vi "_TCP Msg Read.vi"(7 "RT":bool, 8 "error in":errorcluster, 10 "timeout ms (10000)":i32=10000, 11 "connection ID":refnum<k5>) -> (0 "error out":errorcluster, 1 "Read Timeout":bool, 2 "Packet Info":T1={"Packet Signature"="", "Sequence Number"=0, "Command"=enum."xml Set LC Input Logic", "Data Message Size"=0, "Data Message Size"="", "Data Message"="", "Error Message Size"=0, "Error Message Size"="", "Error Message"="", "Checksum"=0, "Error Message"={"status"=FALSE, "code"=0, "source"=""}, "Command ID"=""}, 3 "connection ID out":refnum<k5>)   [LabVIEW 2015]
doc: "Reads an incoming package of data from a remote host via TCP/IP. This VI parses the package and extracts the data name and type as described in the meta data.\n\nFor the package to be parsed correctly, the meta data must be consistent in both the sender and the receiver. The data is packaged based on the existing meta data on the sender. Inconsistent meta data will result in inconsistent data parsing.\nUse the \"Read Meta\" and \"Write Meta\" VIs to ensure that both client and server have the same meta data.\n\nThe data is returned as a string. It is the responsibility of the user to cast it to the appropriate type before usage."
uses:
  Types/TCP Packet Info.ctl
  Types/_RT Command.ctl
  Types/TCP Packet Parsing State Machine.ctl
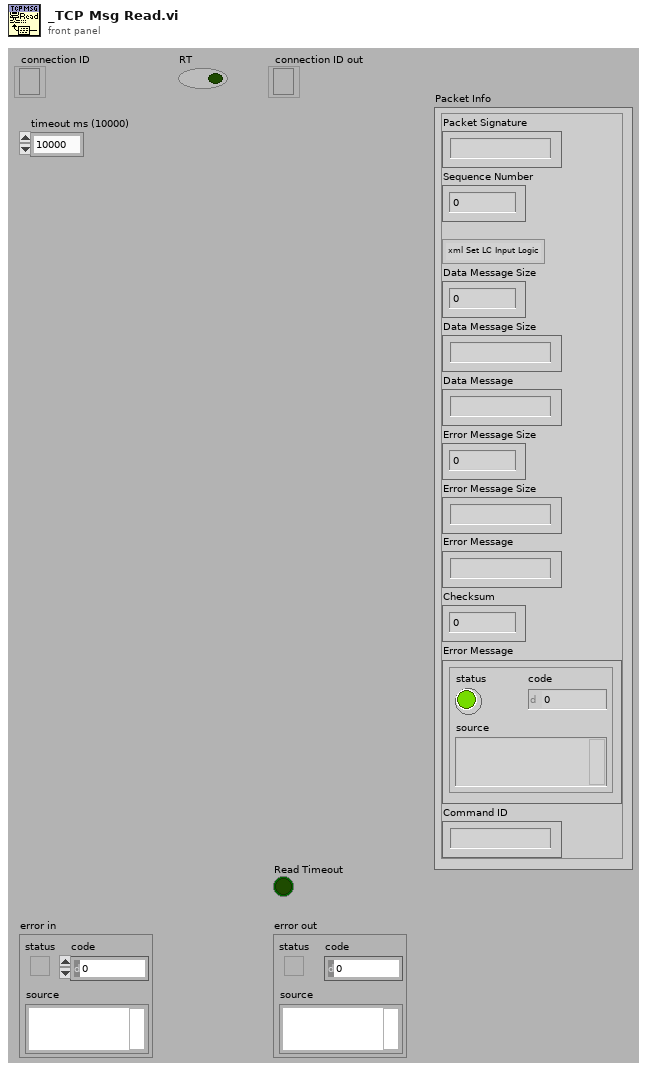
[diagram p1: front panel]
types:
  T1 = typedef "TCP Packet Info.ctl" = cluster{"Packet Signature":string, "Sequence Number":i32, "Command":T2, "Data Message Size":u32, "Data Message Size":string, "Data Message":string, "Error Message Size":u32, "Error Message Size":string, "Error Message":string, "Checksum":u32, "Error Message":errorcluster, "Command ID":string}
  T2 = typedef "_RT Command.ctl" = enum16{"xml Start Run", "xml Start Actual Run", "xml Stop Run", "xml Runtime Update", "xml Get Status", "xml Get Table", "xml Set Table", "xml Get Configuration", "xml System Status", "xml Set LC Input Logic", "xml Get Data", "xml Get Info", "Start", "StartActualRun", "Stop", "Runtime Update", "Get Data", "Get Info", "Get Status", "Get Param", "Get Config", "Get Table", "Read ADC", "Set Oscillator", "Update Config", "Update Table", "Set All Pol", "Set Pol and DC", "Set Max Mass", "Toggle RP", "Toggle EL", "Set PIC", "Initialize Turbo", "Send Turbo Comm", "Close Turbo", "P1", "P2", "P3", "Send Serial", "Set LC Out", "Get LC In", "Read VAC", "Test Table", "Toggle Power", "Get Startup", "Set Startup", "Get ADC Table", "Set ADC Table", "Get Brief Status", "Get Detail Status", "Auxiliary Update", "Set CC Logics", "Set CC Input Logics", "Ignore Error", "invalid"}
  T3 = typedef "TCP Packet Parsing State Machine.ctl" = enum16{"Packet Signature", "Sequence Number", "Command ID", "Data Message Size", "Data Message", "Error Message Size", "Error Message", "Checksum", "Invalid Packet Structure"}
  T4 = enum16{"big-endian, network order", "native, host order", "little-endian"}
  T5 = enum16{"Standard", "Buffered", "CRLF", "Immediate"}
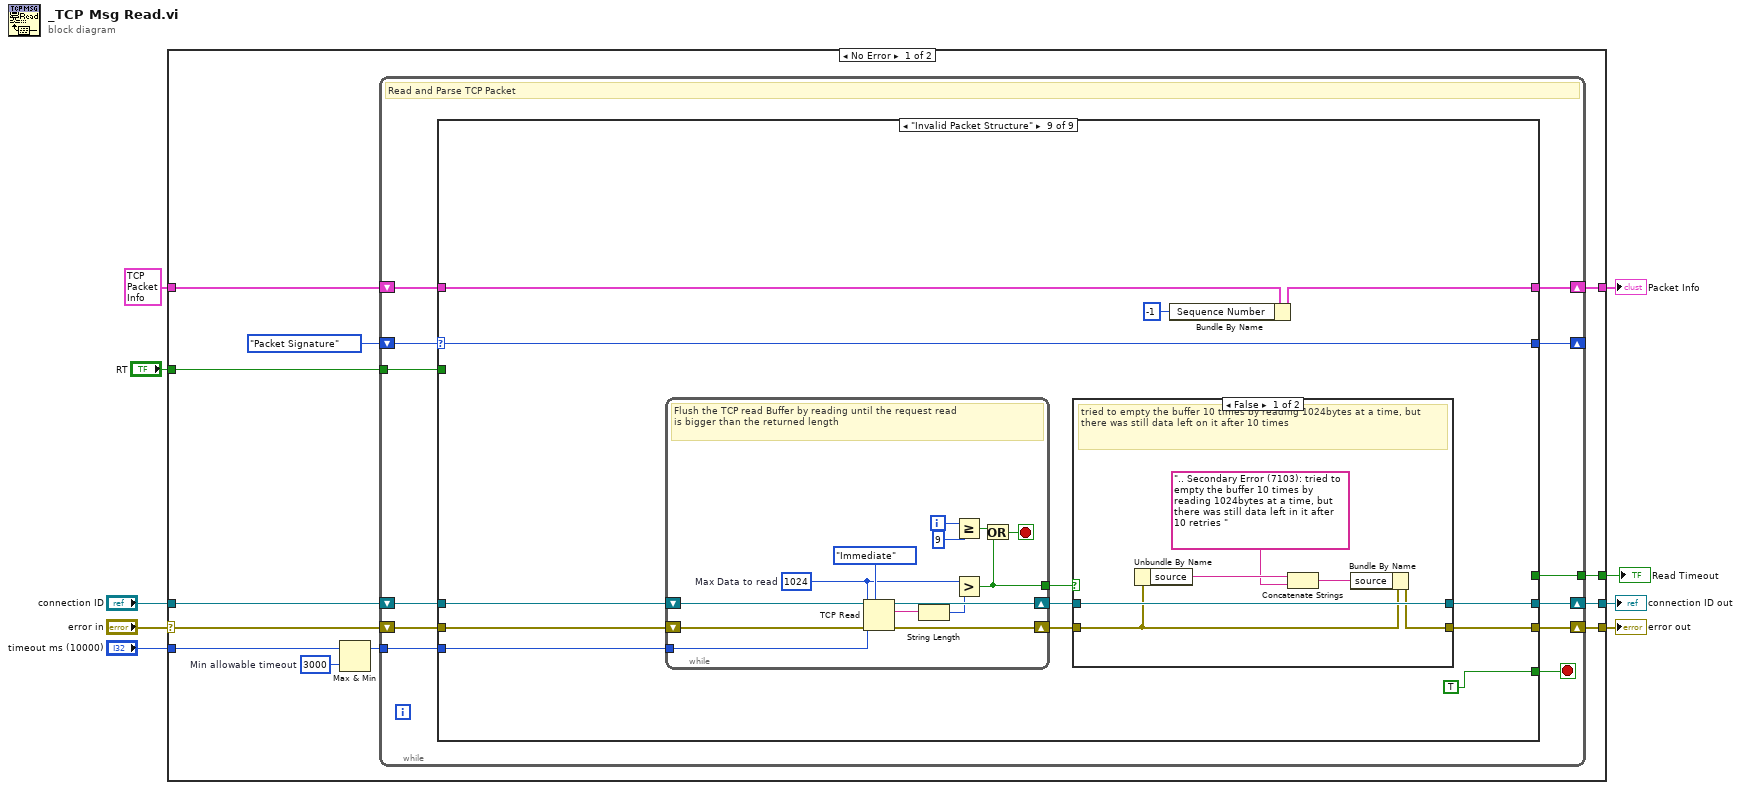
[diagram p0: block diagram]
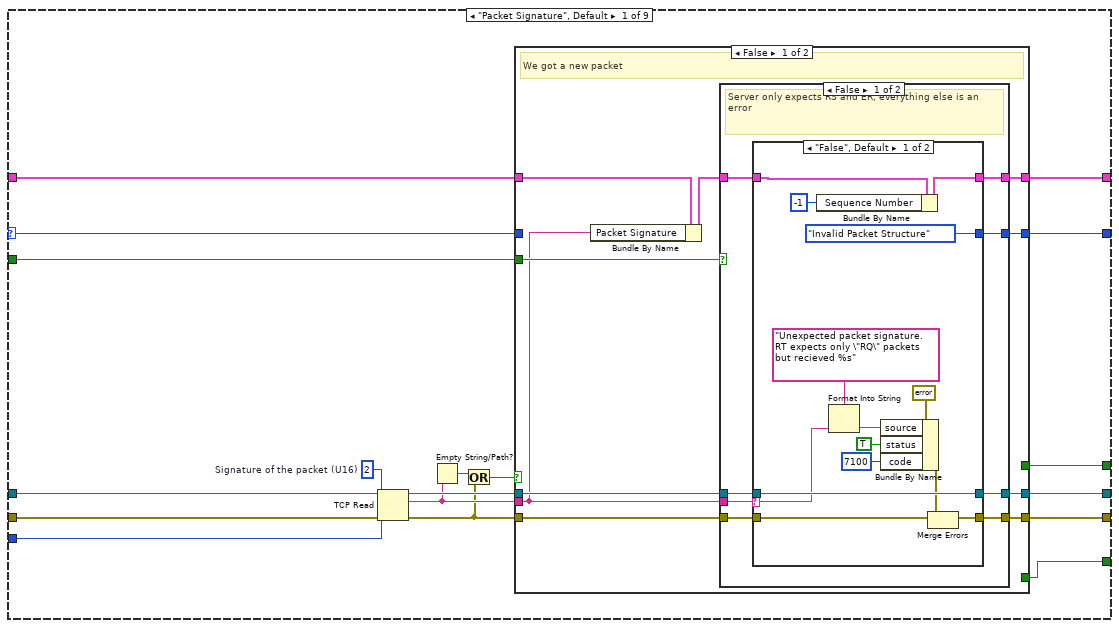
[diagram p2: hidden frame]
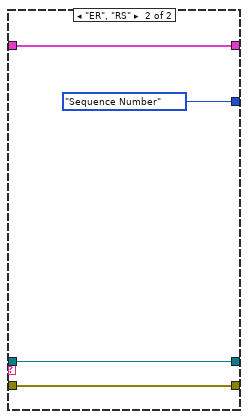
[diagram p3: hidden frame]
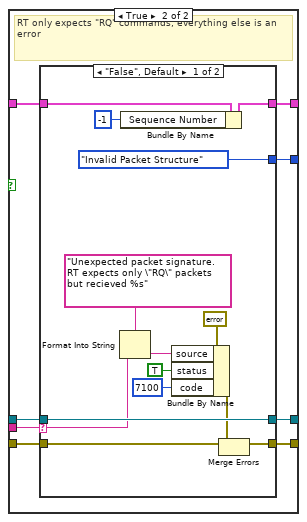
[diagram p4: hidden frame]
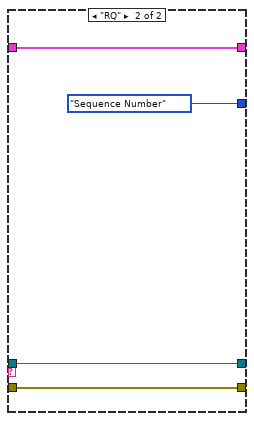
[diagram p5: hidden frame]
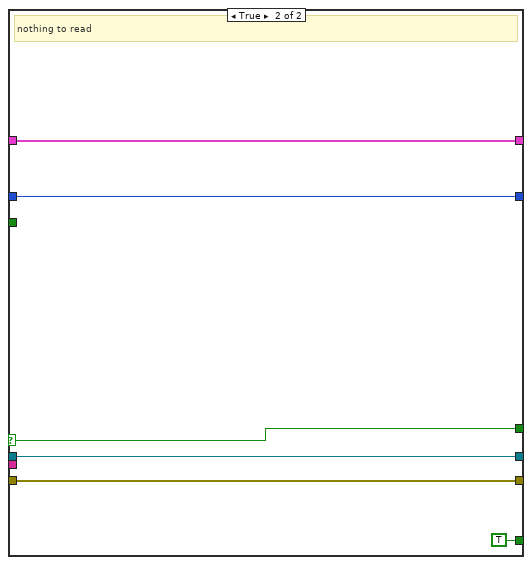
[diagram p6: hidden frame]
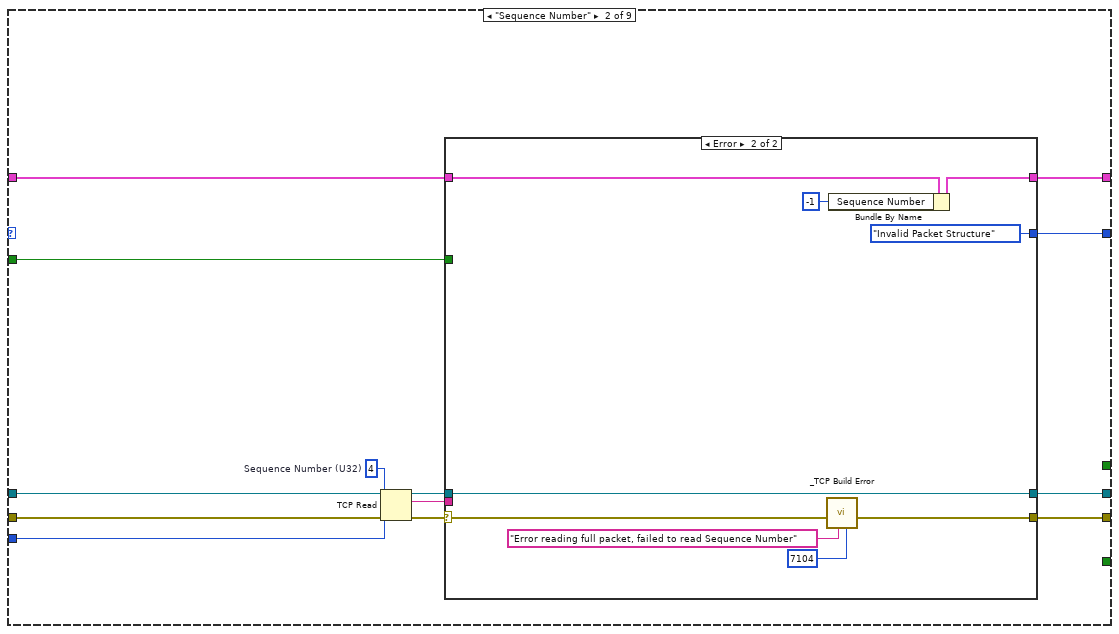
[diagram p7: hidden frame]
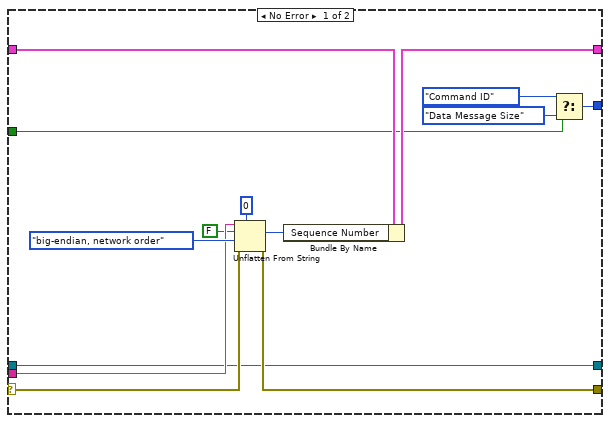
[diagram p8: hidden frame]
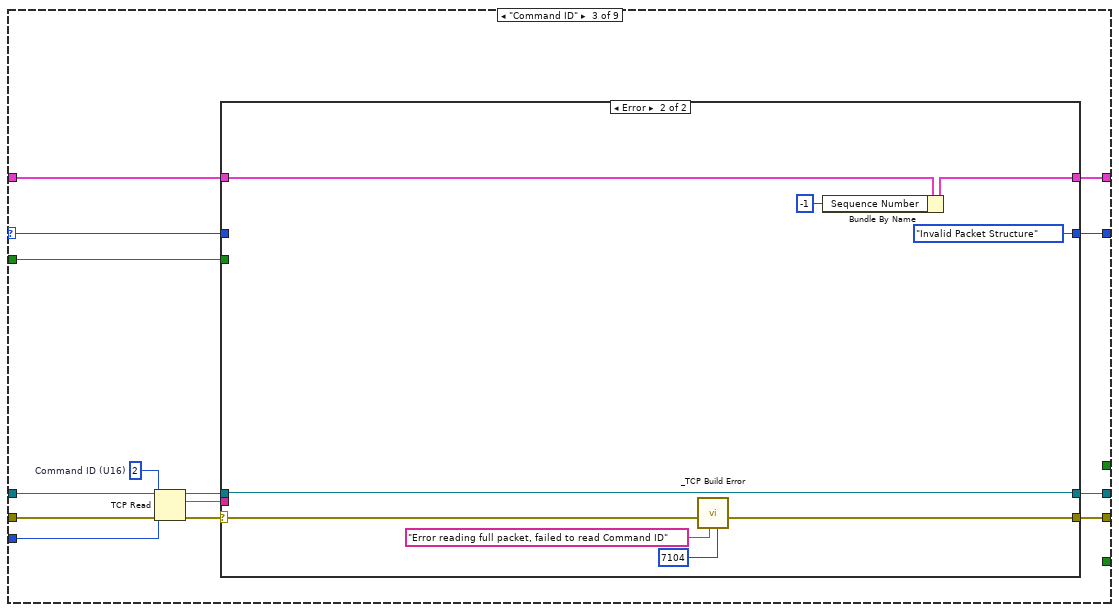
[diagram p9: hidden frame]
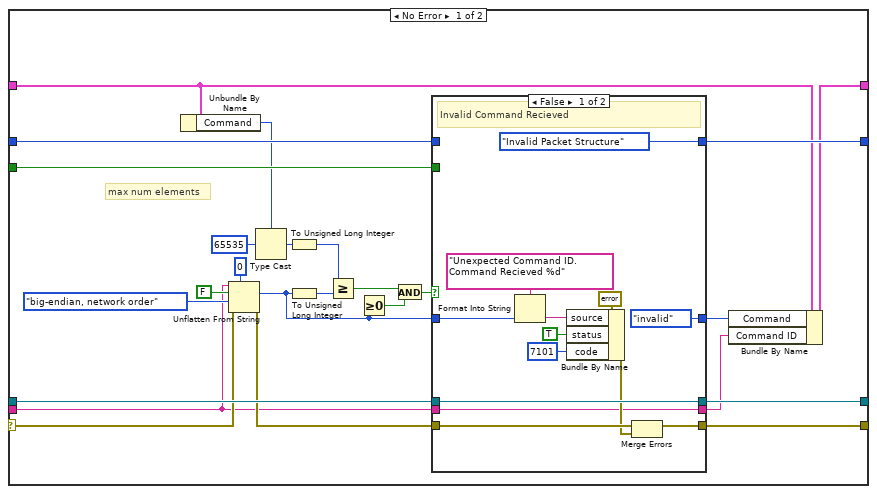
[diagram p10: hidden frame]
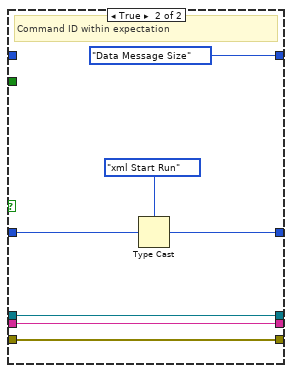
[diagram p11: hidden frame]
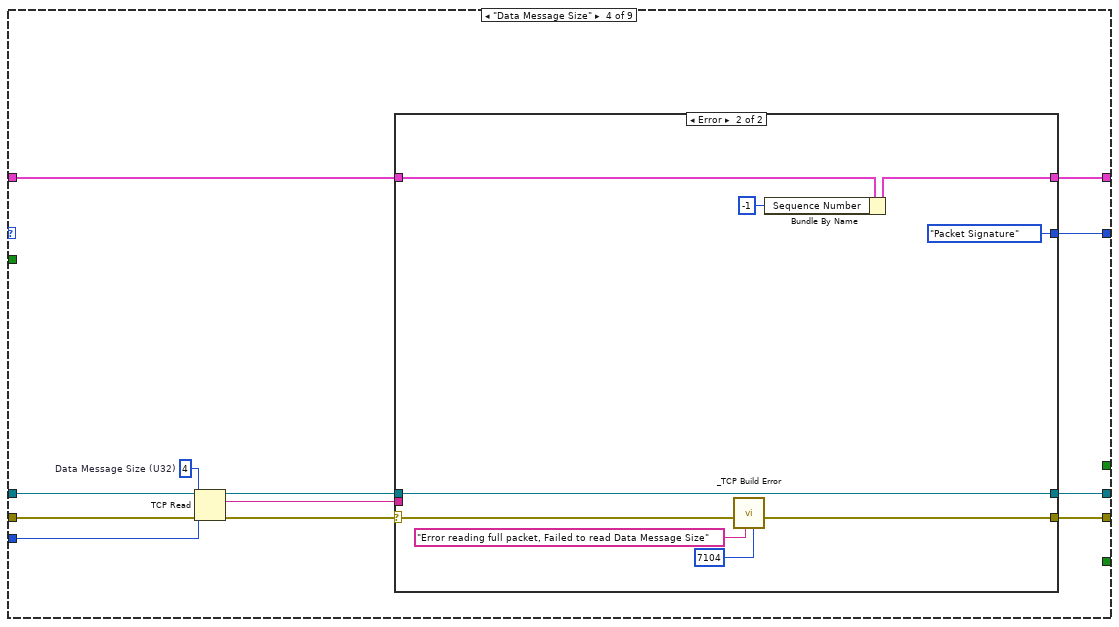
[diagram p12: hidden frame]
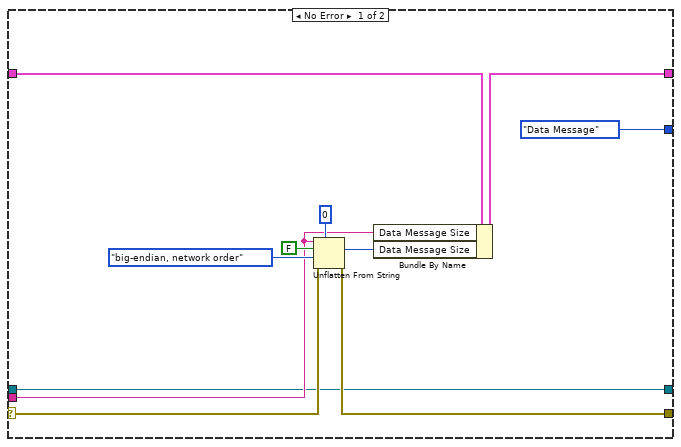
[diagram p13: hidden frame]
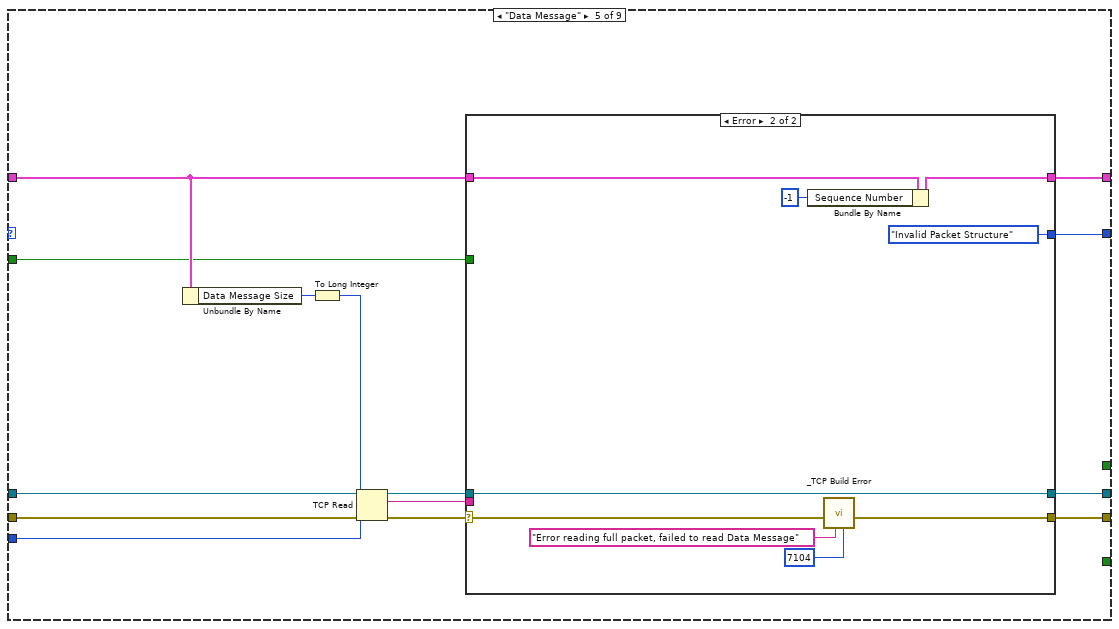
[diagram p14: hidden frame]
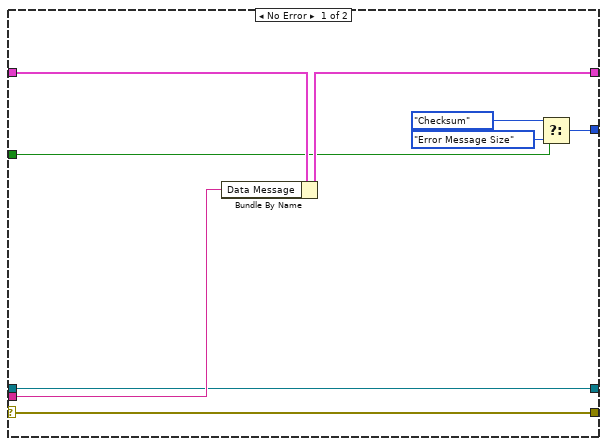
[diagram p15: hidden frame]
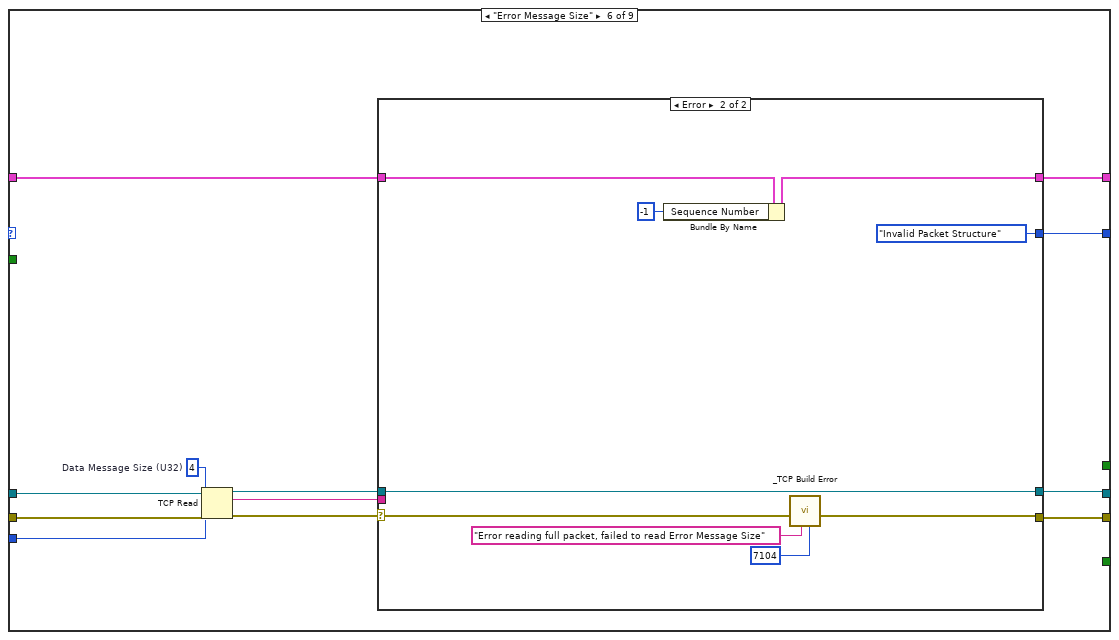
[diagram p16: hidden frame]
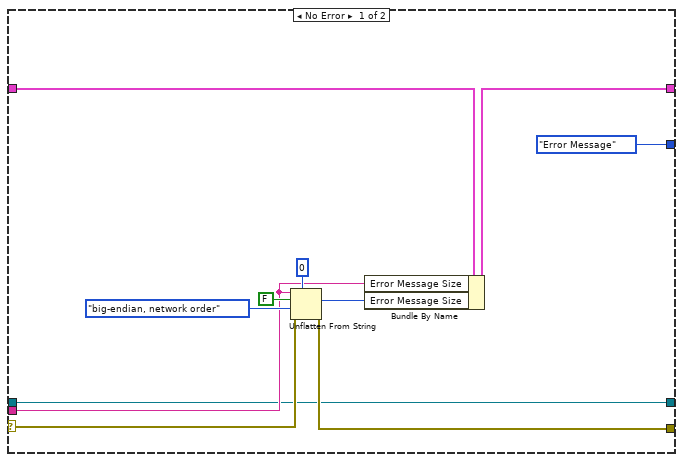
[diagram p17: hidden frame]
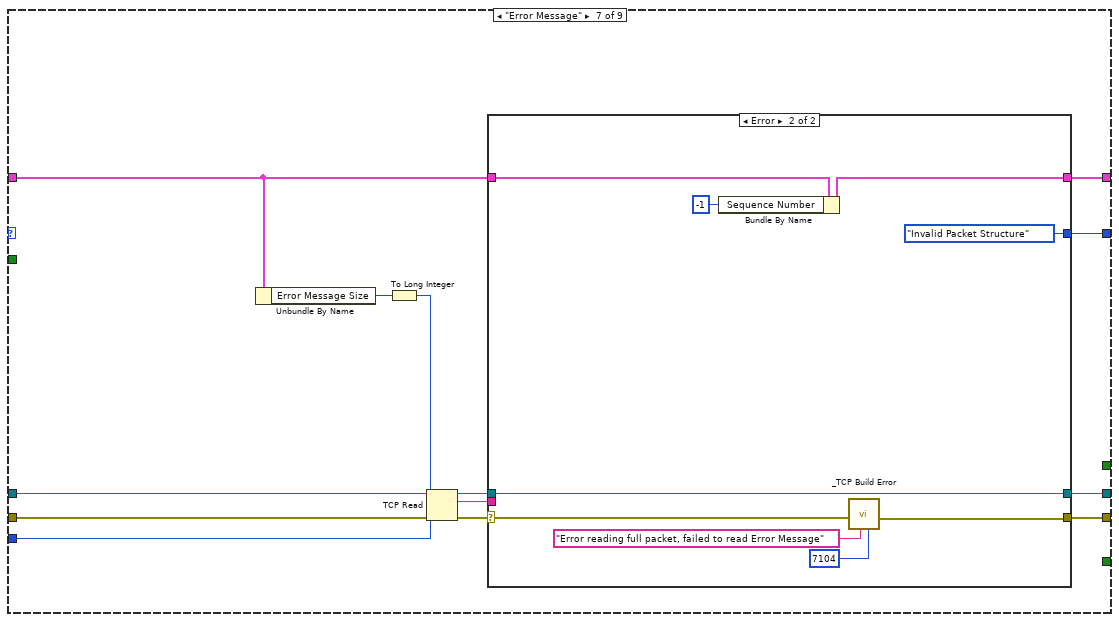
[diagram p18: hidden frame]
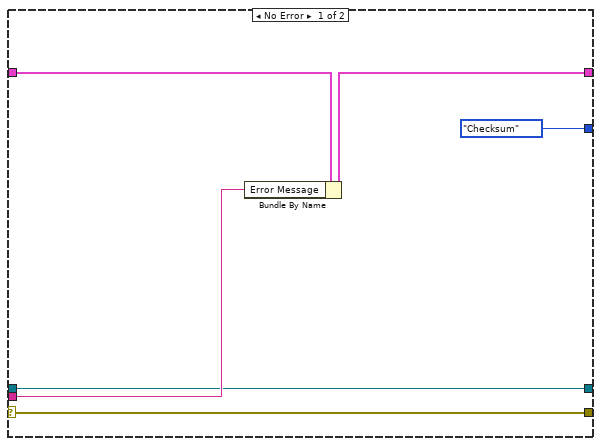
[diagram p19: hidden frame]
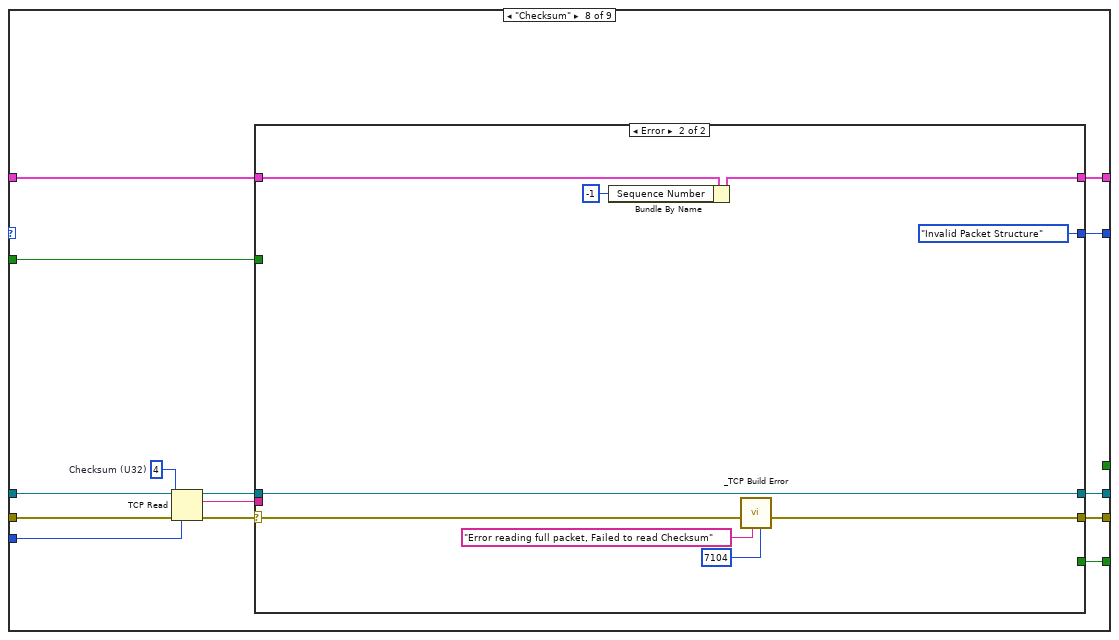
[diagram p20: hidden frame]
diagram:
  n1 = case shown="No Error" "error in" {
    selector: "error in" -> [w19 w453]
    tunnel: T1 {"Packet Signature"="", "Sequence Number"=0, "Command"=enum."xml Set LC Input Logic", "Data Message Size"=0, "Data Message Size"="", "Data Message"="", "Error Message Size"=0, "Error Message Size"="", "Error Message"="", "Checksum"=0, "Error Message"={"status"=FALSE, "code"=0, "source"=""}, "Command ID"=""} ("Packet Info") -> [w21 w452]
    tunnel: "connection ID" -> [w20 w454]
    tunnel: "timeout ms (10000)" -> [w18 _]
    tunnel: "RT" -> [w17 _]
    tunnel: [w16 w454] -> w5
    tunnel: [w15 w453] -> w4
    tunnel: [w14 w452] -> w3
    tunnel: [w10 _] -> w1
    frame No Error {
      w12 = 3000  # Min allowable timeout
      n2 = Max & Min(x=w18, y=w12) -> (max(x,y)=w11:i32)  [unwired: 1 out]
      n3 = while {
        shift-right: [w32] -> w14
        shift-left: w21 -> [w33]
        shift-right: [w27] -> w16
        shift-left: w20 -> [w31]
        shift-right: [w28] -> w15
        shift-left: w19 -> [w30]
        tunnel: w11 -> [w29]
        tunnel: w17 -> [w26]
        shift-right: [w25] -> _
        shift-left: TCP_Packet_Parsing_State_Machine."Packet Signature" ("Packet Structure") -> [w23]
        tunnel: [w22] -> w10
        stop <- w24 stop-if-true
        # "Read and Parse TCP Packet"
        n4 = case shown="\"Invalid Packet Structure\"" w23 {
          selector: w23 -> [w39 _ w164 _ _ _ _ _ w428]
          tunnel: w33 -> [w41 w132 w159 w231 w264 w295 w326 w355 w418]
          tunnel: [w43 w127 w161 w230 w263 w294 w325 w357 w417] -> w32
          tunnel: w31 -> [w50 w130 w167 w233 w268 w297 w328 w361 w426]
          tunnel: w30 -> [w49 w129 w166 w234 w269 w298 w329 w359 w427]
          tunnel: w29 -> [w47 w128 w165 w232 w267 w296 w327 w360 w425]
          tunnel: [w45 w122 w157 w227 w259 w291 w321 w352 w420] -> w28
          tunnel: [w44 w121 w162 w225 w256 w288 w323 w354 w422] -> w27
          tunnel: w26 -> [w46 w126 w160 _ w260 _ _ w348 _]
          tunnel: [w42 w125 w163 w229 w261 w293 w324 w356 w428] -> w25
          tunnel: [w38 _ _ _ _ _ _ w351 TRUE] -> w24
          tunnel: [w37 _ _ _ _ _ _ _ _] -> w22
          frame "Packet Signature", Default {
            w51 = 2  # Signature of the packet (U16)
            # "Packet Header"
            n5 = TCP Read(connection ID=w50, bytes to read=w51, error in (no error)=w49, 9:w47) -> (connection ID out=w48:refnum<k5>, data out=w40:string, error out=w34:errorcluster)  [unwired: 1 out]
            n6 = Empty String/Path?(string/path=w40) -> (empty?=w36:bool)
            n7 = Or(x=w36, y=w34) -> (x .or. y?=w35:bool)
            n8 = case shown="False" w35 {
              selector: w35 -> [_ w114]
              tunnel: w48 -> [w61 w117]
              tunnel: w34 -> [w60 w116]
              tunnel: w46 -> [w59 _]
              tunnel: [w58 w116] -> w45
              tunnel: [w57 w117] -> w44
              tunnel: [w56 w119] -> w43
              tunnel: [w55 w118] -> w42
              tunnel: w41 -> [w54 w119]
              tunnel: w40 -> [w52 _]
              tunnel: w39 -> [_ w118]
              tunnel: [_ TRUE] -> w38
              tunnel: [_ w114] -> w37
              frame False {
                # "We got a new packet"
                n9 = Bundle By Name(cluster=w54, "Packet Signature"=w52) -> (w53:T1)
                n10 = case shown="False" w59 {
                  tunnel: w52 -> [w68 w90]
                  tunnel: w61 -> [w67 w95]
                  tunnel: w60 -> [w69 w94]
                  tunnel: [w66 w93] -> w57
                  tunnel: [w65 w92] -> w58
                  tunnel: w53 -> [w62 w88]
                  tunnel: [w63 w89] -> w56
                  tunnel: [w64 w91] -> w55
                  frame False {
                    # "Server only expects RS and ER, everything else is an error"
                    n11 = case shown="\"False\", Default" w68 {
                      selector: w68 -> [w73 _]
                      tunnel: w69 -> [w75 w86]
                      tunnel: w67 -> [w83 w87]
                      tunnel: [w83 w87] -> w66
                      tunnel: [w76 w86] -> w65
                      tunnel: [TCP_Packet_Parsing_State_Machine."Invalid Packet Structure" ("Packet Structure") TCP_Packet_Parsing_State_Machine."Sequence Number" ("Packet Structure")] -> w64
                      tunnel: [w70 w84] -> w63
                      tunnel: w62 -> [w71 w84]
                      frame "False", Default {
                        n12 = Bundle By Name(cluster=w71, "Sequence Number"=-1) -> (w70:T1)
                        n13 = Format Into String(format string="Unexpected packet signature. RT expects only \"RQ\" packets but recieved %s" ("source"), w73) -> (resulting string=w78:string)  [unwired: 2 in, 1 out]
                        n14 = Bundle By Name(cluster=errorcluster {"status"=FALSE, "code"=0, "source"=""} ("error IO"), "source"=w78, "status"=TRUE, "code"=7100) -> (w77:errorcluster)
                        n15 = Merge Errors(w75, w77) -> (w76:errorcluster)
                      }
                      frame "ER", "RS" {
                      }
                    }
                  }
                  frame True {
                    # "RT only expects \"RQ\" commands, everything else is an error"
                    n16 = case shown="\"False\", Default" w90 {
                      selector: w90 -> [w104 _]
                      tunnel: w95 -> [w109 w113]
                      tunnel: w94 -> [w101 w112]
                      tunnel: [w109 w113] -> w93
                      tunnel: [w100 w112] -> w92
                      tunnel: [TCP_Packet_Parsing_State_Machine."Invalid Packet Structure" ("Packet Structure") TCP_Packet_Parsing_State_Machine."Sequence Number" ("Packet Structure")] -> w91
                      tunnel: [w97 w110] -> w89
                      tunnel: w88 -> [w98 w110]
                      frame "False", Default {
                        n17 = Format Into String(format string="Unexpected packet signature. RT expects only \"RQ\" packets but recieved %s" ("source"), w104) -> (resulting string=w103:string)  [unwired: 2 in, 1 out]
                        n18 = Bundle By Name(cluster=w98, "Sequence Number"=-1) -> (w97:T1)
                        n19 = Bundle By Name(cluster=errorcluster {"status"=FALSE, "code"=0, "source"=""} ("error IO"), "source"=w103, "status"=TRUE, "code"=7100) -> (w102:errorcluster)
                        n20 = Merge Errors(w101, w102) -> (w100:errorcluster)
                      }
                      frame "RQ" {
                        # "\"RQ\""
                      }
                    }
                  }
                }
              }
              frame True {
                # "nothing to read"
              }
            }
          }
          frame "Sequence Number" {
            w131 = 4  # Sequence Number (U32)
            n21 = TCP Read(connection ID=w130, bytes to read=w131, error in (no error)=w129, 9:w128) -> (connection ID out=w120:refnum<k5>, data out=w123:string, error out=w124:errorcluster)  [unwired: 1 out]
            n22 = case shown="Error" w124 {
              selector: w124 -> [w140 w153]
              tunnel: w132 -> [w146 w148]
              tunnel: [w145 w147] -> w127
              tunnel: w126 -> [w144 _]
              tunnel: [w142 TCP_Packet_Parsing_State_Machine."Invalid Packet Structure" ("f")] -> w125
              tunnel: w123 -> [w136 _]
              tunnel: [w134 w152] -> w122
              tunnel: [w133 w155] -> w121
              tunnel: w120 -> [w133 w155]
              frame No Error {
                n23 = Unflatten From String(type=0, binary string=w136, data includes array or string size? (T)=FALSE, byte order (0:big-endian, network order)=T4."big-endian, network order", error in (no error)=w140) -> (value=w137:i32, error out=w134:errorcluster)  [unwired: 1 out]
                n24 = Bundle By Name(cluster=w146, "Sequence Number"=w137) -> (w145:T1)
                n25 = Select(t=TCP_Packet_Parsing_State_Machine."Command ID" ("Packet Structure"), s=w144, f=TCP_Packet_Parsing_State_Machine."Data Message Size") -> (s? t:f=w142:T3)
              }
              frame Error {
                n26 = call "_TCP Build Error.vi"("code"=7104, "Error"="Error reading full packet, failed to read Sequence Number", "error in (no error)"=w153) -> ("error out"=w152:errorcluster)  [unwired: 8 in]
                n27 = Bundle By Name(cluster=w148, "Sequence Number"=-1) -> (w147:T1)
              }
            }
          }
          frame "Command ID" {
            w168 = 2  # Command ID (U16)
            n28 = TCP Read(connection ID=w167, bytes to read=w168, error in (no error)=w166, 9:w165) -> (connection ID out=w169:refnum<k5>, data out=w156:string, error out=w158:errorcluster)  [unwired: 1 out]
            n29 = case shown="Error" w158 {
              selector: w158 -> [w175 w221]
              tunnel: w169 -> [w190 w220]
              tunnel: w164 -> [w186 _]
              tunnel: [w185 TCP_Packet_Parsing_State_Machine."Invalid Packet Structure" ("Packet Structure")] -> w163
              tunnel: [w184 w220] -> w162
              tunnel: [w183 w215] -> w161
              tunnel: w160 -> [w181 _]
              tunnel: w159 -> [w180 w216]
              tunnel: [w172 w219] -> w157
              tunnel: w156 -> [w170 _]
              frame No Error {
                # "max num elements"
                n30 = Unbundle By Name(w180) -> ("Command"=w179:T2)
                n31 = Unflatten From String(type=u16 0, binary string=w170, data includes array or string size? (T)=FALSE, byte order (0:big-endian, network order)=T4."big-endian, network order", error in (no error)=w175) -> (value=w173:u16, error out=w174:errorcluster)  [unwired: 1 out]
                n32 = Type Cast(type=w179, x=u16 65535 ("default value 1")) -> (*(type *) &x=w189:T2)
                n33 = To Unsigned Long Integer(number=w189) -> (unsigned 32bit integer=w187:u32)
                n34 = To Unsigned Long Integer(number=w173) -> (unsigned 32bit integer=w191:u32)
                n35 = Greater Or Equal?(x=w187, y=w191) -> (x >= y?=w192:bool)
                n36 = Greater Or Equal To 0?(x=w173) -> (x >= 0?=w194:bool)
                n37 = And(x=w192, y=w194) -> (x .and. y?=w193:bool)
                n38 = case shown="False" w193 {
                  tunnel: [w198 w214] -> w172
                  tunnel: w174 -> [w200 w214]
                  tunnel: [w207 w213] -> w184
                  tunnel: w190 -> [w207 w213]
                  tunnel: w173 -> [w201 w212]
                  tunnel: [_RT_Command."invalid" ("Command") w211] -> w182
                  tunnel: w186 -> [_ _]
                  tunnel: [TCP_Packet_Parsing_State_Machine."Invalid Packet Structure" ("Packet Structure") TCP_Packet_Parsing_State_Machine."Data Message Size" ("Packet Structure")] -> w185
                  tunnel: w181 -> [_ _]
                  tunnel: [w195 w208] -> w171
                  tunnel: w170 -> [w195 w208]
                  frame False {
                    # "Invalid Command Recieved"
                    n39 = Format Into String(format string="Unexpected Command ID. Command Recieved %d" ("source"), w201) -> (resulting string=w202:string)  [unwired: 2 in, 1 out]
                    n40 = Bundle By Name(cluster=errorcluster {"status"=FALSE, "code"=0, "source"=""} ("error IO"), "source"=w202, "status"=TRUE, "code"=7101) -> (w199:errorcluster)
                    n41 = Merge Errors(w200, w199) -> (w198:errorcluster)
                  }
                  frame True {
                    # "Command ID within expectation"
                    n42 = Type Cast(type=_RT_Command."xml Start Run" ("Command"), x=w212) -> (*(type *) &x=w211:T2)
                  }
                }
                n43 = Bundle By Name(cluster=w180, "Command"=w182, "Command ID"=w171) -> (w183:T1)
              }
              frame Error {
                n44 = call "_TCP Build Error.vi"("code"=7104, "Error"="Error reading full packet, failed to read Command ID", "error in (no error)"=w221) -> ("error out"=w219:errorcluster)  [unwired: 8 in]
                n45 = Bundle By Name(cluster=w216, "Sequence Number"=-1) -> (w215:T1)
              }
            }
          }
          frame "Data Message Size" {
            w235 = 4  # Data Message Size (U32)
            n46 = TCP Read(connection ID=w233, bytes to read=w235, error in (no error)=w234, 9:w232) -> (connection ID out=w224:refnum<k5>, data out=w226:string, error out=w228:errorcluster)  [unwired: 1 out]
            n47 = case shown="Error" w228 {
              selector: w228 -> [w241 w252]
              tunnel: w231 -> [w246 w248]
              tunnel: [w245 w247] -> w230
              tunnel: [TCP_Packet_Parsing_State_Machine."Data Message" ("Packet Structure") TCP_Packet_Parsing_State_Machine."Packet Signature" ("Packet Structure")] -> w229
              tunnel: [w238 w251] -> w227
              tunnel: w226 -> [w237 _]
              tunnel: [w236 w255] -> w225
              tunnel: w224 -> [w236 w255]
              frame No Error {
                n48 = Unflatten From String(type=u32 0 ("default value 1"), binary string=w237, data includes array or string size? (T)=FALSE, byte order (0:big-endian, network order)=T4."big-endian, network order", error in (no error)=w241) -> (value=w239:u32, error out=w238:errorcluster)  [unwired: 1 out]
                n49 = Bundle By Name(cluster=w246, "Data Message Size"=w237, "Data Message Size"=w239) -> (w245:T1)
              }
              frame Error {
                n50 = call "_TCP Build Error.vi"("code"=7104, "Error"="Error reading full packet, Failed to read Data Message Size", "error in (no error)"=w252) -> ("error out"=w251:errorcluster)  [unwired: 8 in]
                n51 = Bundle By Name(cluster=w248, "Sequence Number"=-1) -> (w247:T1)
              }
            }
          }
          frame "Data Message" {
            n52 = Unbundle By Name(w264) -> ("Data Message Size"=w266:u32)
            n53 = To Long Integer(number=w266) -> (32bit integer=w265:i32)
            n54 = TCP Read(connection ID=w268, bytes to read=w265, error in (no error)=w269, 9:w267) -> (connection ID out=w257:refnum<k5>, data out=w262:string, error out=w258:errorcluster)  [unwired: 1 out]
            n55 = case shown="Error" w258 {
              selector: w258 -> [w271 w283]
              tunnel: w264 -> [w278 w280]
              tunnel: [w277 w279] -> w263
              tunnel: w262 -> [w276 _]
              tunnel: [w273 TCP_Packet_Parsing_State_Machine."Invalid Packet Structure" ("f")] -> w261
              tunnel: w260 -> [w272 _]
              tunnel: [w271 w282] -> w259
              tunnel: w257 -> [w270 w287]
              tunnel: [w270 w287] -> w256
              frame No Error {
                n56 = Bundle By Name(cluster=w278, "Data Message"=w276) -> (w277:T1)
                n57 = Select(t=TCP_Packet_Parsing_State_Machine."Checksum" ("Packet Structure"), s=w272, f=TCP_Packet_Parsing_State_Machine."Error Message Size") -> (s? t:f=w273:T3)
              }
              frame Error {
                n58 = Bundle By Name(cluster=w280, "Sequence Number"=-1) -> (w279:T1)
                n59 = call "_TCP Build Error.vi"("code"=7104, "Error"="Error reading full packet, failed to read Data Message", "error in (no error)"=w283) -> ("error out"=w282:errorcluster)  [unwired: 8 in]
              }
            }
          }
          frame "Error Message Size" {
            w299 = 4  # Data Message Size (U32)
            n60 = TCP Read(connection ID=w297, bytes to read=w299, error in (no error)=w298, 9:w296) -> (connection ID out=w289:refnum<k5>, data out=w290:string, error out=w292:errorcluster)  [unwired: 1 out]
            n61 = case shown="Error" w292 {
              selector: w292 -> [w305 w315]
              tunnel: w295 -> [w310 w312]
              tunnel: [w309 w311] -> w294
              tunnel: [TCP_Packet_Parsing_State_Machine."Error Message" ("Packet Structure") TCP_Packet_Parsing_State_Machine."Invalid Packet Structure" ("Packet Structure")] -> w293
              tunnel: [w302 w314] -> w291
              tunnel: w290 -> [w301 _]
              tunnel: w289 -> [w300 w318]
              tunnel: [w300 w318] -> w288
              frame No Error {
                n62 = Unflatten From String(type=u32 0 ("Error Message Size"), binary string=w301, data includes array or string size? (T)=FALSE, byte order (0:big-endian, network order)=T4."big-endian, network order", error in (no error)=w305) -> (value=w303:u32, error out=w302:errorcluster)  [unwired: 1 out]
                n63 = Bundle By Name(cluster=w310, "Error Message Size"=w301, "Error Message Size"=w303) -> (w309:T1)
              }
              frame Error {
                n64 = Bundle By Name(cluster=w312, "Sequence Number"=-1) -> (w311:T1)
                n65 = call "_TCP Build Error.vi"("code"=7104, "Error"="Error reading full packet, failed to read Error Message Size", "error in (no error)"=w315) -> ("error out"=w314:errorcluster)  [unwired: 8 in]
              }
            }
          }
          frame "Error Message" {
            n66 = Unbundle By Name(w326) -> ("Error Message Size"=w332:u32)
            n67 = To Long Integer(number=w332) -> (32bit integer=w331:i32)
            n68 = TCP Read(connection ID=w328, bytes to read=w331, error in (no error)=w329, 9:w327) -> (connection ID out=w322:refnum<k5>, data out=w330:string, error out=w320:errorcluster)  [unwired: 1 out]
            n69 = case shown="Error" w320 {
              selector: w320 -> [w334 w345]
              tunnel: w330 -> [w338 _]
              tunnel: w326 -> [w337 w340]
              tunnel: [w336 w339] -> w325
              tunnel: [TCP_Packet_Parsing_State_Machine."Checksum" ("Packet Structure") TCP_Packet_Parsing_State_Machine."Invalid Packet Structure" ("Packet Structure")] -> w324
              tunnel: [w333 w347] -> w323
              tunnel: w322 -> [w333 w347]
              tunnel: [w334 w344] -> w321
              frame No Error {
                n70 = Bundle By Name(cluster=w337, "Error Message"=w338) -> (w336:T1)
              }
              frame Error {
                n71 = Bundle By Name(cluster=w340, "Sequence Number"=-1) -> (w339:T1)
                n72 = call "_TCP Build Error.vi"("code"=7104, "Error"="Error reading full packet, failed to read Error Message", "error in (no error)"=w345) -> ("error out"=w344:errorcluster)  [unwired: 8 in]
              }
            }
          }
          frame "Checksum" {
            w358 = 4  # Checksum (U32)
            n73 = TCP Read(connection ID=w361, bytes to read=w358, error in (no error)=w359, 9:w360) -> (connection ID out=w353:refnum<k5>, data out=w349:string, error out=w350:errorcluster)  [unwired: 1 out]
            n74 = case shown="Error" w350 {
              selector: w350 -> [w367 w411]
              tunnel: [w379 w409] -> w357
              tunnel: [w378 TCP_Packet_Parsing_State_Machine."Invalid Packet Structure" ("Packet Structure")] -> w356
              tunnel: w355 -> [w377 w414]
              tunnel: [w374 w412] -> w354
              tunnel: w353 -> [w373 w412]
              tunnel: [w372 w410] -> w352
              tunnel: [w371 _] -> w351
              tunnel: w349 -> [w365 _]
              tunnel: w348 -> [w362 _]
              frame No Error {
                n75 = case shown="False" w362 {
                  tunnel: w377 -> [w385 w388]
                  tunnel: [w384 w387] -> w376
                  frame False {
                    n76 = Unbundle By Name(w385) -> ("Data Message Size"=w383:string, "Data Message"=w382:string, "Error Message Size"=w381:string, "Error Message"=w380:string)
                    n77 = Concatenate Strings(w383, w382, w381, w380) -> (w384:string)
                  }
                  frame True {
                    n78 = Unbundle By Name(w388) -> ("Command ID"=w386:string, "Data Message Size"=w390:string, "Data Message"=w389:string)
                    n79 = Concatenate Strings(w386, w390, w389) -> (w387:string)
                  }
                }
                n80 = Unflatten From String(type=u32 0 ("Checksum"), binary string=w365, data includes array or string size? (T)=FALSE, byte order (0:big-endian, network order)=T4."big-endian, network order", error in (no error)=w367) -> (value=w363:u32, error out=w366:errorcluster)  [unwired: 1 out]
                n81 = call "_Calculate Check Sum.vi"("Stream"=w376) -> ("Checksum"=w370:u16)
                n82 = Equal?(x=w370, y=w363) -> (x = y?=w375:bool)
                n83 = Bundle By Name(cluster=w377, "Checksum"=w363) -> (w379:T1)
                n84 = case shown="False" w375 {
                  tunnel: [TCP_Packet_Parsing_State_Machine."Invalid Packet Structure" ("Packet Structure") TCP_Packet_Parsing_State_Machine."Packet Signature" ("Packet Structure")] -> w378
                  tunnel: [w402 w406] -> w374
                  tunnel: w373 -> [w402 w406]
                  tunnel: [w394 w405] -> w372
                  tunnel: w366 -> [w396 w405]
                  tunnel: [TRUE TRUE] -> w371
                  tunnel: w370 -> [w393 _]
                  tunnel: w363 -> [w392 _]
                  frame False {
                    # "Checksum Invalid"
                    n85 = Format Into String(format string="Checksum is Invalid. Recieved %d, expected %d" ("source"), w392, w393) -> (resulting string=w397:string)  [unwired: 2 in, 1 out]
                    n86 = Bundle By Name(cluster=errorcluster {"status"=FALSE, "code"=0, "source"=""} ("error IO"), "source"=w397, "status"=TRUE, "code"=7102) -> (w395:errorcluster)
                    n87 = Merge Errors(w396, w395) -> (w394:errorcluster)
                  }
                  frame True {
                    # "Valid Checksum"
                  }
                }
              }
              frame Error {
                n88 = Bundle By Name(cluster=w414, "Sequence Number"=-1) -> (w409:T1)
                n89 = call "_TCP Build Error.vi"("code"=7104, "Error"="Error reading full packet, Failed to read Checksum", "error in (no error)"=w411) -> ("error out"=w410:errorcluster)  [unwired: 8 in]
              }
            }
          }
          frame "Invalid Packet Structure" {
            n90 = while {
              tunnel: w425 -> [w447]
              shift-right: [w448] -> w421
              shift-left: w427 -> [w451]
              shift-right: [w449] -> w423
              shift-left: w426 -> [w450]
              tunnel: [w438] -> w424
              i -> [w445]
              stop <- w442 stop-if-true
              w440 = 1024  # Max Data to read
              # "Flush the TCP read Buffer by reading until the request read\nis bigger than the returned length"
              n91 = TCP Read(connection ID=w450, bytes to read=w440, error in (no error)=w451, 7:T5."Immediate" ("mode (standard)"), 9:w447) -> (connection ID out=w449:refnum<k5>, data out=w441:string, error out=w448:errorcluster)
              n92 = String Length(string=w441) -> (length=w439:i32)
              n93 = Greater Or Equal?(x=w445, y=9) -> (x >= y?=w443:bool)
              n94 = Greater?(x=w440, y=w439) -> (0:w438:bool)
              n95 = Or(x=w443, y=w438) -> (x .or. y?=w442:bool)
            }
            n96 = case shown="False" w424 {
              tunnel: w423 -> [w435 w437]
              tunnel: [w435 w437] -> w422
              tunnel: w421 -> [w433 w436]
              tunnel: [w434 w436] -> w420
              frame False {
                # "tried to empty the buffer 10 times by reading 1024bytes at a time, but there was still data left on it after 10 times"
                n97 = Unbundle By Name(w433) -> ("source"=w432:string)
                n98 = Concatenate Strings(w432, ".. Secondary Error (7103): tried to empty the buffer 10 times by reading 1024bytes at a time, but there was still data left in it after 10 retries " ("string")) -> (w431:string)
                n99 = Bundle By Name(cluster=w433, "source"=w431) -> (w434:errorcluster)
              }
              frame True {
                # "Flush was successful"
              }
            }
            n100 = Bundle By Name(cluster=w418, "Sequence Number"=-1) -> (w417:T1)
          }
        }
      }
    }
    frame Error {
    }
  }
  "error out" <- w4
  "connection ID out" <- w5
  "Packet Info" <- w3
  "Read Timeout" <- w1
